vi "331AB_lucrarea iii.7.vi"() -> ()   [LabVIEW 2014]
panel:
  out "Temperatura medie":dbl(slide) scale=0.0..100.0
  out "comanda incalzitor":bool
  in  "stop":bool
  in  "Limita inferioara":dbl
  in  "Limita superioara":dbl
  out "Valoare convertita [V]":u16
  out "Temperatura curenta":u16
  out "Grafic temperaturi":T1(graph)
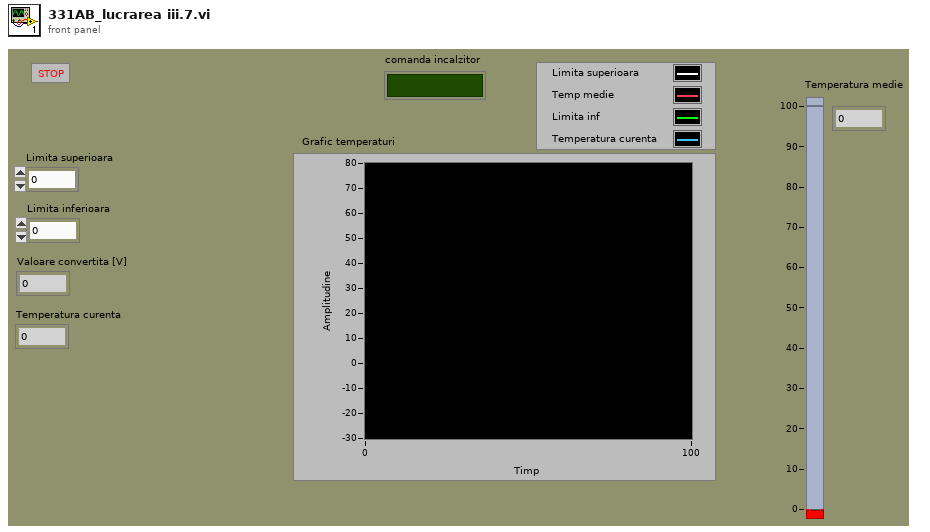
[diagram p1: front panel]
types:
  T1 = cluster{"Limita superioara":dbl, "Numeric":dbl, "Limita inferioara":dbl, dbl}
  T2 = cluster{"Limita superioara":dbl, dbl, "Limita inferioara":dbl, dbl}
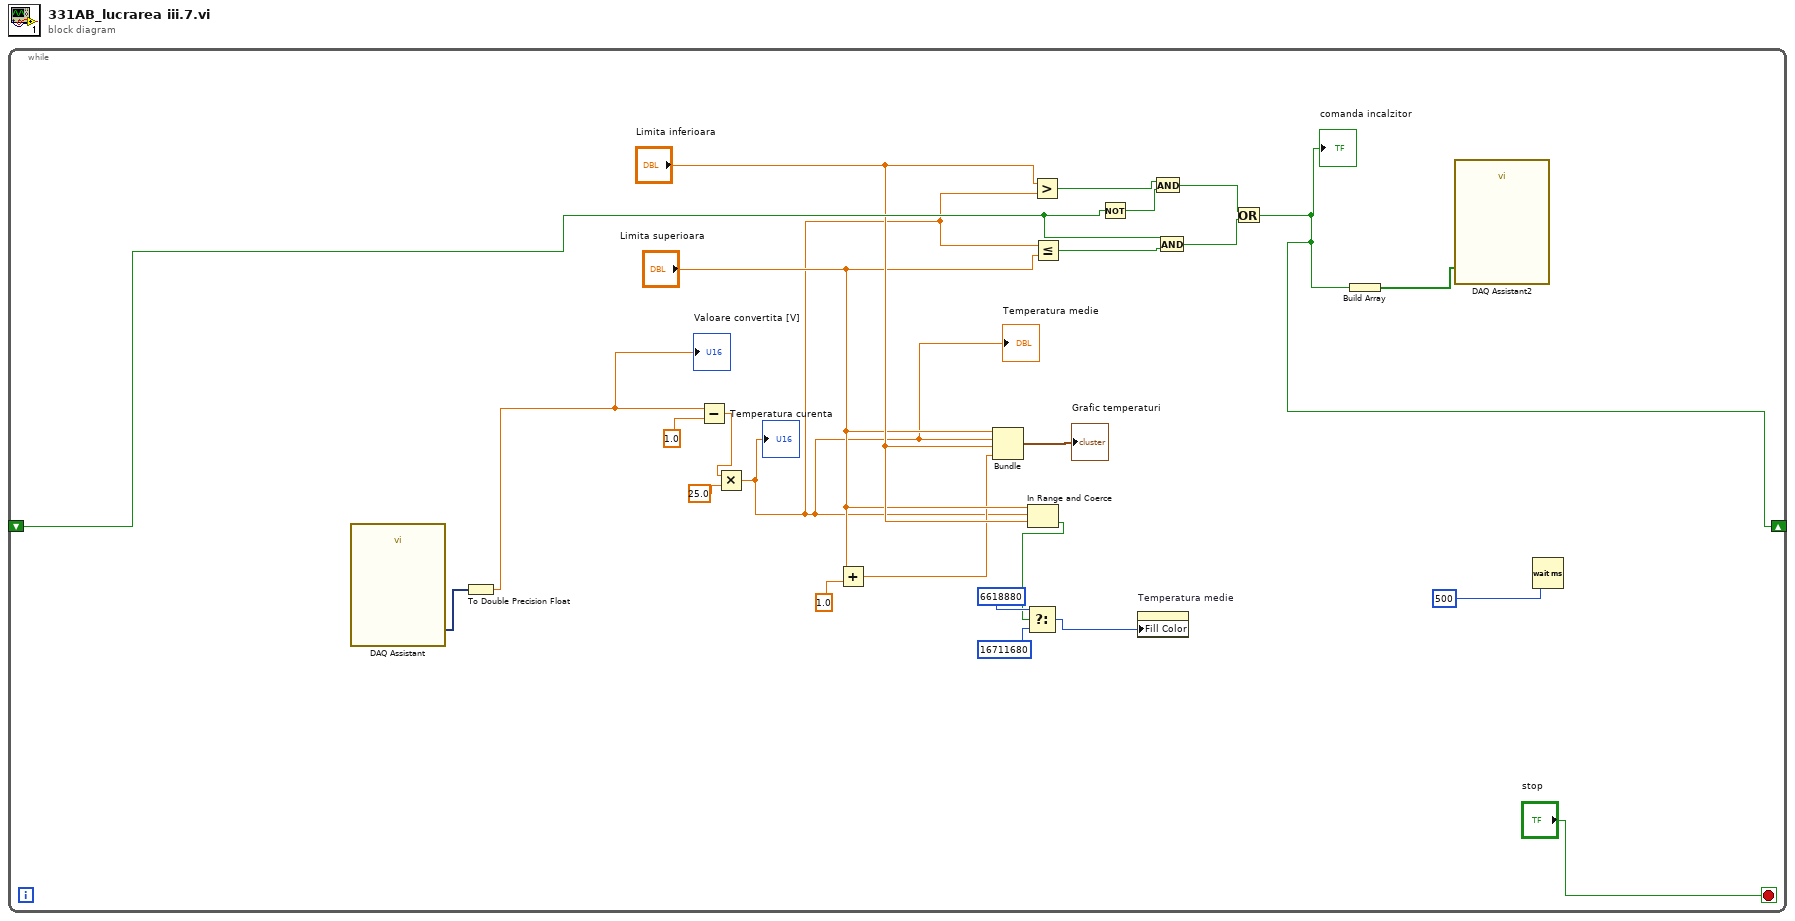
[diagram p0: block diagram]
diagram:
  n1 = while {
    shift-right: [w13] -> _
    shift-left: _ -> [w14]
    stop <- "stop" stop-if-true
    n2 = call "DAQ Assistant"() -> ("data"=w24:dynamicdata)  [unwired: 17 in, 2 out]
    n3 = To Double Precision Float(number=w24) -> (double precision float=w3:dbl)
    "Valoare convertita [V]" <- w3
    n4 = Subtract(x=w3, y=1.0) -> (x-y=w21:dbl)
    n5 = Multiply(x=w21, y=25.0) -> (x*y=w1:dbl)
    "Temperatura curenta" <- w1
    "Temperatura medie" <- w1
    n6 = Add(x="Limita superioara", y=1.0) -> (x+y=w4:dbl)
    n7 = Bundle("Limita superioara"="Limita superioara", w1, "Limita inferioara"="Limita inferioara", w4) -> (→"Grafic temperaturi":T2)  [unwired: 1 in]
    n8 = In Range and Coerce(upper limit="Limita superioara", x=w1, lower limit="Limita inferioara") -> (In Range?=w9:bool)  [unwired: 1 out]
    n9 = Select(t=6618880, s=w9, f=16711680) -> (s? t:f=w2:i32)
    n10 = Greater?(x="Limita inferioara", y=w1) -> (0:w20:bool)
    n11 = Less Or Equal?(x=w1, y="Limita superioara") -> (x <= y?=w17:bool)
    n12 = Not(x=w14) -> (.not. x?=w15:bool)
    n13 = property on="Temperatura medie" class="Slide (strict)"("Fill Color"=w2) -> ()  [unwired: 2 in, 2 out]
    n14 = And(x=w20, y=w15) -> (x .and. y?=w19:bool)
    n15 = And(x=w14, y=w17) -> (x .and. y?=w16:bool)
    n16 = Or(x=w19, y=w16) -> (x .or. y?=w13:bool)
    "comanda incalzitor" <- w13
    n17 = Build Array(w13) -> (w18:bool[])
    n18 = call "DAQ Assistant2"("data"=w18) -> ()  [unwired: 17 in, 2 out]
    n19 = Wait (ms)(milliseconds to wait=500) -> ()  [unwired: 1 out]
  }
